vi "Build.vi"(9 "XYZTheta":dbl[](array[numeric]), 10 "Pattern Coordinates":dbl[][](array[numeric]), 11 "C4 Dispense in":refnum<class "Iterative Dispense.lvclass">) -> (1 "Starting Coordinates":dbl[](array[numeric]), 3 "C4 Dispense out":refnum<class "Iterative Dispense.lvclass">)   [LabVIEW 2016, in "Iterative Dispense.lvclass"]
uses:
  Iterative Dispense.lvclass
  Iterative Dispense.lvclass/Iterative Dispense.ctl
  <vilib>/Analysis/coordinate.llb/2D Cartesian Coordinate Rotation (Array).vi
  <vilib>/Analysis/NI_AALPro.lvlib
panel:
  out "array w/ subset deleted":dbl[][][](array[numeric])
  out "deleted portion":dbl[][](array[numeric])
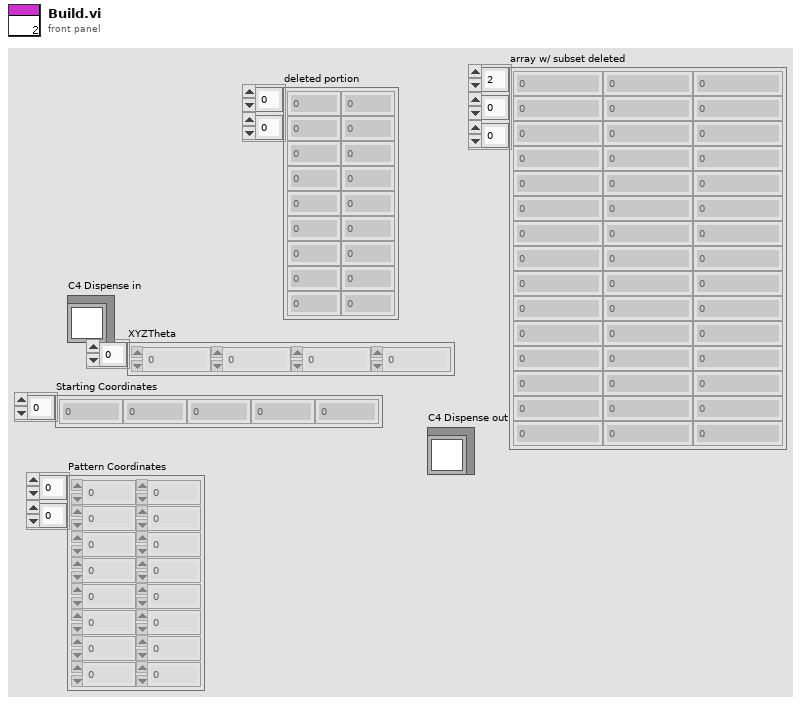
[diagram p1: front panel]
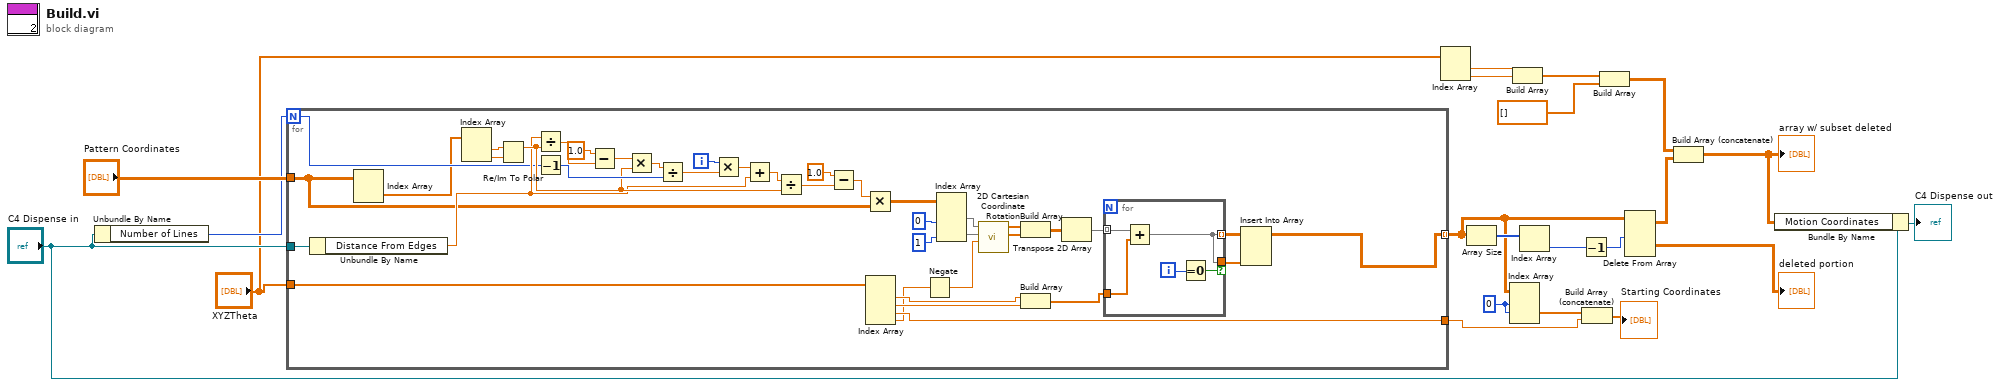
[diagram p0: block diagram]
diagram:
  w21 = 0 ("disabled index (page)")
  n1 = Unbundle By Name("C4 Dispense in") -> ("Number of Lines"=w16:i32)
  n2 = for {
    N: w16 -> [w37]
    tunnel: [w22] -> w8 mode=indexing
    tunnel: "XYZTheta" -> [w23]
    tunnel: "C4 Dispense in" -> [w42]
    tunnel: "Pattern Coordinates" -> [w31]
    tunnel: [w36] -> w19
    i -> [w55]
    n3 = Unbundle By Name(w42) -> ("Distance From Edges"=w41:dbl)
    n4 = Index Array(array=w31) -> (element=w30:dbl[])  [unwired: 2 in]
    n5 = Index Array(array=w30) -> (element #1=w29:dbl, element #2=w28:dbl)  [unwired: 2 in]
    n6 = Re/Im To Polar(2:w28, 3:w29) -> (1:w43:dbl)  [unwired: 1 out]
    n7 = Divide(x=w41, y=w43) -> (x/y=w49:dbl)
    n8 = Decrement(x=w37) -> (x-1=w45:i32)
    n9 = Subtract(x=1.0, y=w49) -> (x-y=w47:dbl)
    n10 = Multiply(x=w47, y=w43) -> (x*y=w46:dbl)
    n11 = Divide(x=w46, y=w45) -> (x/y=w44:dbl)
    n12 = Multiply(x=w55, y=w44) -> (x*y=w60:dbl)
    n13 = Add(x=w60, y=w41) -> (x+y=w59:dbl)
    n14 = Divide(x=w59, y=w43) -> (x/y=w58:dbl)
    n15 = Subtract(x=1.0, y=w58) -> (x-y=w50:dbl)
    n16 = Multiply(x=w50, y=w31) -> (x*y=w56:dbl[][])
    n17 = Index Array(array=w23) -> (element #1=w40:dbl, element #2=w39:dbl, element #3=w36:dbl, element #4=w25:dbl)  [unwired: 4 in]
    n18 = Negate(x=w25) -> (-x=w24:dbl)
    n19 = Index Array(array=w56, index (col) #1=0 ("disabled index (col)"), index (col) #2=1 ("index (col)")) -> (element #1=w35:dbl[], element #2=w34:dbl[])  [unwired: 2 in]
    n20 = call-poly <vilib>:"2D Cartesian Coordinate Rotation.vi"("theta"=w24, "Y"=w34, "X"=w35) -> ("Y Out"=w54:dbl[], "X Out"=w53:dbl[])  [unwired: 6 in, 1 out]
    n21 = Build Array(w53, w54) -> (w27:dbl[][])
    n22 = Build Array(w40, w39) -> (w38:dbl[])
    n23 = Transpose 2D Array(2D array=w27) -> (transposed array=w26:dbl[][])
    n24 = for {
      tunnel: w38 -> [w65]
      tunnel: w26 -> [w64] mode=indexing
      tunnel: [w61] -> w33 mode=indexing
      tunnel: [w61] -> w32 if=w62
      i -> [w63]
      n25 = Add(x=w64, y=w65) -> (x+y=w61:dbl[])
      n26 = Equal To 0?(x=w63) -> (x = 0?=w62:bool)
    }
    n27 = Insert Into Array(array=w33, new element=w32) -> (w22:dbl[][])  [unwired: 2 in]
  }
  n28 = Index Array(array="XYZTheta") -> (element #1=w3:dbl, element #2=w2:dbl)  [unwired: 2 in]
  n29 = Array Size(array=w8) -> (size(s)=w13:i32[])
  n30 = Index Array "Index Array"(array=w8, index (dim 0)=w21, index (dim 1)=w21) -> (element=w20:dbl[])  [unwired: 1 in]
  n31 = Build Array(w3, w2) -> (w1:dbl[])
  n32 = Index Array(array=w13) -> (element=w11:i32)  [unwired: 1 in]
  n33 = Decrement(x=w11) -> (x-1=w10:i32)
  n34 = Build Array (concatenate)(w20, w19) -> (→"Starting Coordinates":dbl[])
  n35 = Build Array(w1, dbl[] [] ("element")) -> (w9:dbl[][])
  n36 = Delete From Array "Delete From Array"(array=w8, index (dim 0)=w10) -> (deleted portion=→"deleted portion":dbl[][], array with subset deleted=w6:dbl[][][])  [unwired: 3 in]
  n37 = Build Array (concatenate)(w9, w6) -> (w5:dbl[][][])
  "array w/ subset deleted" <- w5
  n38 = Bundle By Name(cluster="C4 Dispense in", "Motion Coordinates"=w5) -> (→"C4 Dispense out":refnum<class "Iterative Dispense.lvclass">)
